vi "OAT Output Trigger Event (waveform).vi"(0 "signal in":waveform(dbl), 1 "trigger on":T1(ring), 2 "reset? (F)":bool, 5 "upper setpoint":dbl=inf, 7 "lower setpoint":dbl=-inf, 9 "hysteresis":dbl format="%.2p", 11 "error in (no error)":errorcluster) -> (4 "trigger detected?":bool, 15 "error out":errorcluster)   [LabVIEW 2017, in "SoundVib_OAUtility.lvlib"]
doc: "Detects the first level-crossing condition. The <B>upper setpoint</B> and <B>lower setpoint</B> of the threshold and the <B>hysteresis</B> specify the trigger conditions. Wire data to the <B>signal in</B> input to determine the polymorphic instance to use or manually select the instance."
uses:
  <vilib>/addons/Sound and Vibration/Order Analysis/Utility/SoundVib_OAUtility.lvlib
  <vilib>/addons/_NISVFA/_Shared subVIs/Common/svc_Check for Waveform Parameter Continuity (no state).vi
  <vilib>/addons/_NISVFA/_Shared subVIs/Common/svc_Get SV Channel Info.vi
  <vilib>/measure/mamon.llb/Trigger Detection for 1 Channel.vi
  <vilib>/addons/_NISVFA/_Shared subVIs/Common/svc_Engineering Units to Unit Label.vi
  <vilib>/addons/_NISVFA/_Shared subVIs/Common/svc_Unit Label to Engineering Units.vi
  <vilib>/measure/NI_MAPro.lvlib
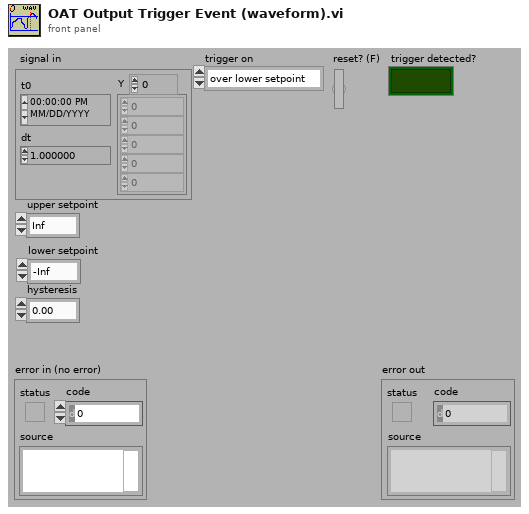
[diagram p1: front panel]
types:
  T1 = enum16{"over lower setpoint", "under upper setpoint", "both"}
  T2 = cluster{"dt":bool, "t0 continuity":bool, "array length":bool, "channel info":bool, "name":bool}
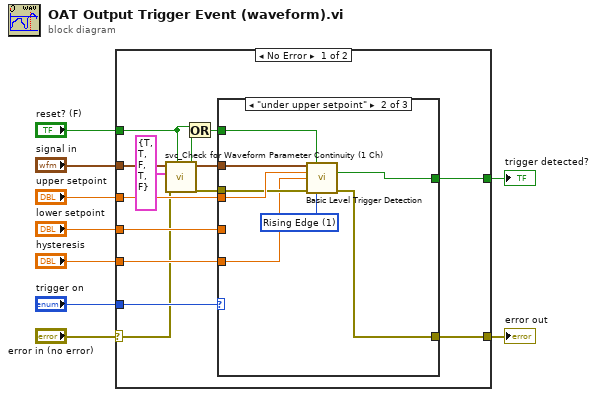
[diagram p0: block diagram]
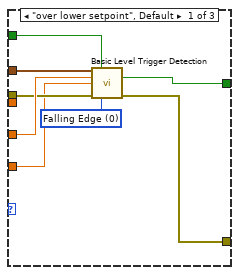
[diagram p2: hidden frame]
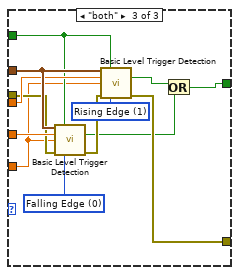
[diagram p3: hidden frame]
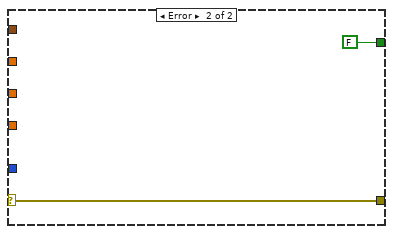
[diagram p4: hidden frame]
diagram:
  n1 = case shown="No Error" "error in (no error)" {
    selector: "error in (no error)" -> [w11 w54]
    tunnel: [w20 w54] -> w8
    tunnel: "trigger on" -> [w23 _]
    tunnel: "signal in" -> [w22 _]
    tunnel: "reset? (F)" -> [w14 _]
    tunnel: "lower setpoint" -> [w21 _]
    tunnel: [w19 FALSE ("trigger detected?")] -> w3
    tunnel: "upper setpoint" -> [w18 _]
    tunnel: "hysteresis" -> [w17 _]
    frame No Error {
      n2 = call <vilib>:"svc_Check for Waveform Parameter Continuity (1 Ch).vi"("restart averaging (F)"=w14, "error in (no error)"=w11, "checks for channel parameter change"=T2 {"dt"=TRUE, "t0 continuity"=TRUE, "array length"=FALSE, "channel info"=TRUE, "name"=FALSE}, "scaled signal [EU]"=w22) -> ("error out"=w10:errorcluster, "waveform parameter changed"=w13:bool, "dup scaled signal [EU]"=w16:waveform(dbl))  [unwired: 2 in, 3 out]
      n3 = Or(x=w14, y=w13) -> (x .or. y?=w15:bool)
      n4 = case shown="\"under upper setpoint\"" w23 {
        tunnel: w16 -> [w31 w39 w52]
        tunnel: w15 -> [w30 w38 w41]
        tunnel: w21 -> [w28 _ w50]
        tunnel: w10 -> [w27 w36 w47]
        tunnel: [w26 w33 w45] -> w20
        tunnel: [w25 w34 w42] -> w19
        tunnel: w18 -> [_ w37 w51]
        tunnel: w17 -> [w24 w32 w40]
        frame "over lower setpoint", Default {
          w29 = u16 0 items=["Falling Edge", "Rising Edge"] ("slope")
          n5 = call-poly <vilib>:"Basic Level Trigger Detection.vi"("signal in"=w31, "reset"=w30, "level"=w28, "hysteresis"=w24, "error in (no error)"=w27, "trigger slope"=w29) -> ("trigger detected?"=w25:bool, "error out"=w26:errorcluster)  [unwired: 7 in, 1 out]
        }
        frame "under upper setpoint" {
          w35 = u16 1 items=["Falling Edge", "Rising Edge"] ("slope")
          n6 = call-poly <vilib>:"Basic Level Trigger Detection.vi"("signal in"=w39, "reset"=w38, "level"=w37, "hysteresis"=w32, "error in (no error)"=w36, "trigger slope"=w35) -> ("trigger detected?"=w34:bool, "error out"=w33:errorcluster)  [unwired: 7 in, 1 out]
        }
        frame "both" {
          w48 = u16 0 items=["Falling Edge", "Rising Edge"] ("slope")
          w49 = u16 1 items=["Falling Edge", "Rising Edge"] ("slope")
          n7 = call-poly <vilib>:"Basic Level Trigger Detection.vi"("signal in"=w52, "reset"=w41, "level"=w50, "hysteresis"=w40, "error in (no error)"=w47, "trigger slope"=w48) -> ("trigger detected?"=w43:bool, "error out"=w46:errorcluster)  [unwired: 7 in, 1 out]
          n8 = call-poly <vilib>:"Basic Level Trigger Detection.vi"("signal in"=w52, "reset"=w41, "level"=w51, "hysteresis"=w40, "error in (no error)"=w46, "trigger slope"=w49) -> ("trigger detected?"=w44:bool, "error out"=w45:errorcluster)  [unwired: 7 in, 1 out]
          n9 = Or(x=w44, y=w43) -> (x .or. y?=w42:bool)
        }
      }
    }
    frame Error {
    }
  }
  "error out" <- w8
  "trigger detected?" <- w3
